vi "Crosshair.vi"(8 "Y":dbl, 9 "X":dbl, 11 "Webcam In":T1) -> (3 "Webcam out":T1)   [LabVIEW 2013]
uses:
  <vilib>/vision/Image Controls.llb/IMAQ Image.ctl
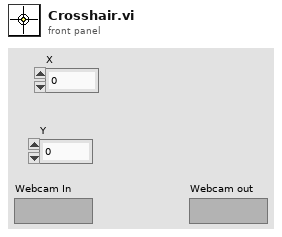
[diagram p1: front panel]
types:
  T1 = typedef "IMAQ Image.ctl" = refnum<image>
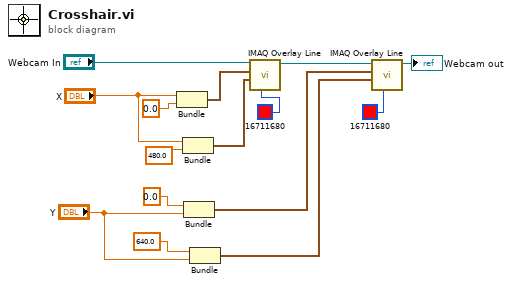
[diagram p0: block diagram]
diagram:
  n1 = Bundle("X"="X", "element"=0.0) -> (w13:cluster{"X":dbl, "element":dbl})  [unwired: 1 in]
  n2 = Bundle("X"="X", "element"=480.0) -> (w10:cluster{"X":dbl, "element":dbl})  [unwired: 1 in]
  n3 = Bundle("element"=0.0, "Y"="Y") -> (w6:cluster{"element":dbl, "Y":dbl})  [unwired: 1 in]
  n4 = Bundle("element"=640.0, "Y"="Y") -> (w5:cluster{"element":dbl, "Y":dbl})  [unwired: 1 in]
  n5 = call "IMAQ Overlay Line"("Color"=u32 16711680, "End Point"=w10, "Start Point"=w13, "Image"="Webcam In") -> ("Image Out"=w4:T1)  [unwired: 6 in, 1 out]
  n6 = call "IMAQ Overlay Line"("Color"=u32 16711680, "End Point"=w5, "Start Point"=w6, "Image"=w4) -> ("Image Out"=→"Webcam out":T1)  [unwired: 6 in, 1 out]
